vi "Button Text Write.vi"(4 "error in (no error)":errorcluster, 5 "Value":string, 6 "Container State":T2, 7 "Display State In":T1) -> (0 "error out":errorcluster, 3 "Display State Out":T1)   [LabVIEW 2009, in "Previous Button (System).xctl"]
uses:
  <vilib>/Navigation Controls/Previous Button System/Previous Button (System).xctl
  <vilib>/_xctls/Container State.ctl
  <vilib>/Navigation Controls/Previous Button System/Previous Button State.ctl
  <vilib>/_xctls/XControlSupport.lvlib
panel:
  # "Replace the Value Control below with a Control of desired type.\nDo not remove this Control or the others from the connector pane.\nDo not change the connector pane pattern.\nThe Value control should always be the third terminal from top on the input side in the connector pane."
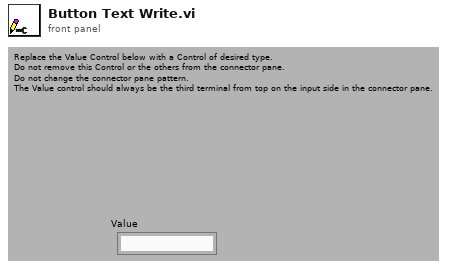
[diagram p1: front panel]
types:
  T1 = typedef "Previous Button (System).xctl/Previous Button State.ctl" = cluster{"Button Text":string}
  T2 = typedef "XControlSupport.lvlib/Container State.ctl" = cluster{"Indicator?":bool, "Run Mode?":bool, " Refnum":refnum<vi>}
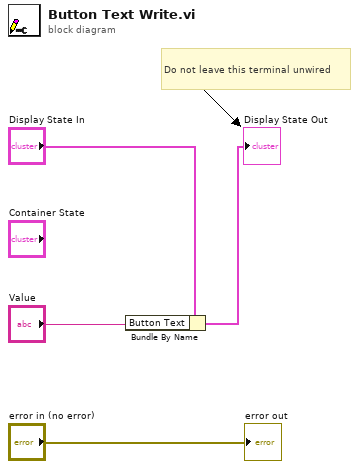
[diagram p0: block diagram]
diagram:
  # "Do not leave this terminal unwired"
  n1 = Bundle By Name(cluster="Display State In", "Button Text"="Value") -> (→"Display State Out":T1)
  "error out" <- "error in (no error)"
